vi "U3 Multiple EI-1050 Example.vi"() -> ()   [LabVIEW 2021]
panel:
  in  "stop":bool
  out "ms per iteration":u32
  out "RH B [%]":dbl format="%.6f"
  out "RH A [%]":dbl format="%.6f"
  out "Temp B [degC]":dbl format="%.6f"
  out "Temp A [degC]":dbl format="%.6f"
  out "Error Message":string
  out "error out":errorcluster
  # "Reads temperature and humidity from a pair of EI-1050 probes:\n\nBoth Probes:\nRed (Power)         FIO6\nBlack (Ground)     GND\nGreen (Data)        FIO4\nWhite (Clock)       FIO5\n\nProbe A:\nBrown (Enable)    FIO7\n\nProbe B:\nBrown (Enable)    DAC0"
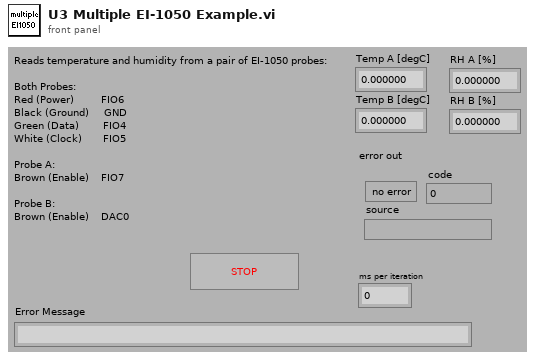
[diagram p1: front panel]
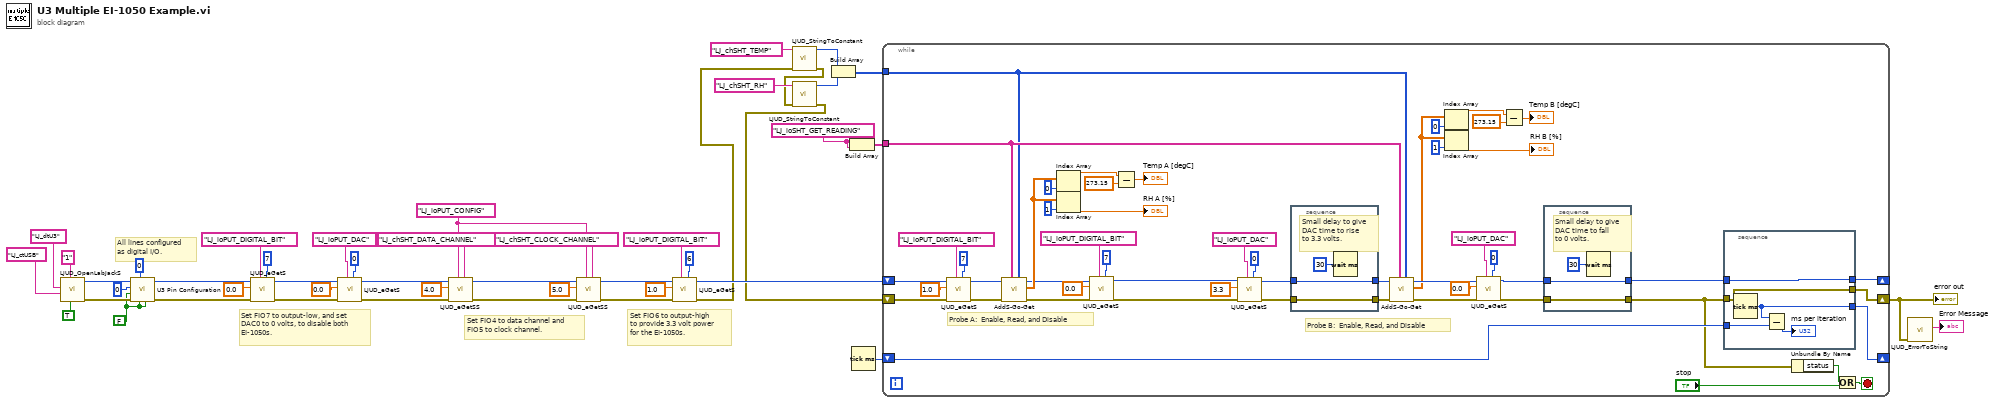
[diagram p0: block diagram]
diagram:
  w3 = "LJ_ioPUT_CONFIG"
  w39 = FALSE ("Enable DAC1")
  w34 = "LJ_ioSHT_GET_READING" ("IOType")
  # "Set FIO4 to data channel and\nFIO5 to clock channel."
  # "Set FIO7 to output-low, and set\nDAC0 to 0 volts, to disable both\nEI-1050s."
  # "Set FIO6 to output-high\nto provide 3.3 volt power\nfor the EI-1050s."
  # "All lines configured\nas digital I/O."
  n1 = call "LJUD_OpenLabJackS.vi"("FirstFound"=TRUE, "Address"="1", "ConnectionType"="LJ_ctUSB", "DeviceType"="LJ_dtU3") -> ("error out"=w41:errorcluster, "Handle"=w42:i32)  [unwired: 5 in, 1 out]
  n2 = call "U3 Pin Configuration.vi"("Enable Counter1"=w39, "Enable Counter0"=w39, "FIO/EIO Analog Enable"=0, "error in"=w41, "Enable DAC1"=w39, "Number of Timers Enabled"=u8 0, "Handle In"=w42) -> ("error out"=w20:errorcluster, "Handle Out"=w21:i32)  [unwired: 3 in]
  n3 = call "LJUD_eGetS.vi"("Channel"=7, "IOType"="LJ_ioPUT_DIGITAL_BIT", "error in"=w20, "Value Write"=0.0, "Handle In"=w21) -> ("error out"=w22:errorcluster, "Handle Out"=w23:i32)  [unwired: 4 in, 1 out]
  n4 = call "LJUD_eGetS.vi"("Channel"=0, "IOType"="LJ_ioPUT_DAC", "error in"=w22, "Value Write"=0.0, "Handle In"=w23) -> ("error out"=w5:errorcluster, "Handle Out"=w7:i32)  [unwired: 4 in, 1 out]
  n5 = call "LJUD_eGetSS.vi"("Channel"="LJ_chSHT_DATA_CHANNEL" ("IOType"), "IOType"=w3, "error in"=w5, "Value Write"=4.0, "Handle In"=w7) -> ("error out"=w11:errorcluster, "Handle Out"=w10:i32)  [unwired: 4 in, 1 out]
  n6 = call "LJUD_eGetSS.vi"("Channel"="LJ_chSHT_CLOCK_CHANNEL" ("IOType"), "IOType"=w3, "error in"=w11, "Value Write"=5.0, "Handle In"=w10) -> ("error out"=w4:errorcluster, "Handle Out"=w6:i32)  [unwired: 4 in, 1 out]
  n7 = call "LJUD_eGetS.vi"("Channel"=6, "IOType"="LJ_ioPUT_DIGITAL_BIT", "error in"=w4, "Value Write"=1.0, "Handle In"=w6) -> ("error out"=w14:errorcluster, "Handle Out"=w16:i32)  [unwired: 4 in, 1 out]
  n8 = call "LJUD_StringToConstant.vi"("error in"=w14, "String"="LJ_chSHT_TEMP") -> ("error out"=w13:errorcluster, "Constant Number"=w33:i32)  [unwired: 8 in]
  n9 = call "LJUD_StringToConstant.vi"("error in"=w13, "String"="LJ_chSHT_RH") -> ("error out"=w12:errorcluster, "Constant Number"=w32:i32)  [unwired: 8 in]
  n10 = Build Array(w33, w32) -> (w18:i32[])
  n11 = Build Array(w34, w34) -> (w19:string[])
  n12 = Tick Count (ms)() -> (millisecond timer value=w17:u32)
  n13 = while {
    shift-left: w17 -> [w59]
    shift-right: [w62] -> _
    shift-left: w16 -> [w63]
    shift-right: [w60] -> _
    shift-left: w12 -> [w64]
    shift-right: [w61] -> w15
    tunnel: w18 -> [w65]
    tunnel: w19 -> [w66]
    stop <- w58 stop-if-true
    # "Probe B:  Enable, Read, and Disable"
    # "Probe A:  Enable, Read, and Disable"
    n14 = call "LJUD_eGetS.vi"("Channel"=7, "IOType"="LJ_ioPUT_DIGITAL_BIT", "error in"=w64, "Value Write"=1.0, "Handle In"=w63) -> ("error out"=w89:errorcluster, "Handle Out"=w90:i32)  [unwired: 4 in, 1 out]
    n15 = call "AddS-Go-Get.vi"("Channels"=w65, "IOTypes"=w66, "error in"=w89, "Handle In"=w90) -> ("error out"=w84:errorcluster, "Values Read"=w98:dbl[], "Handle Out"=w85:i32)  [unwired: 5 in]
    n16 = Index Array(array=w98, index=0 ("Index")) -> (element=w95:dbl)
    n17 = Index Array(array=w98, index=1 ("Index")) -> (element=→"RH A [%]":dbl)
    n18 = call "LJUD_eGetS.vi"("Channel"=7, "IOType"="LJ_ioPUT_DIGITAL_BIT", "error in"=w84, "Value Write"=0.0, "Handle In"=w85) -> ("error out"=w69:errorcluster, "Handle Out"=w70:i32)  [unwired: 4 in, 1 out]
    n19 = Subtract(x=w95, y=273.15) -> (x-y=→"Temp A [degC]":dbl)
    n20 = call "LJUD_eGetS.vi"("Channel"=0, "IOType"="LJ_ioPUT_DAC", "error in"=w69, "Value Write"=3.3, "Handle In"=w70) -> ("error out"=w55:errorcluster, "Handle Out"=w53:i32)  [unwired: 4 in, 1 out]
    n21 = stacked-sequence {
      tunnel: w55 -> [w106]
      tunnel: [w106] -> w54
      tunnel: w53 -> [w105]
      tunnel: [w105] -> w52
      frame #0 {
        # "Small delay to give\nDAC time to rise\nto 3.3 volts."
        n22 = Wait (ms)(milliseconds to wait=u32 30) -> ()  [unwired: 1 out]
      }
    }
    n23 = call "AddS-Go-Get.vi"("Channels"=w65, "IOTypes"=w66, "error in"=w54, "Handle In"=w52) -> ("error out"=w83:errorcluster, "Values Read"=w73:dbl[], "Handle Out"=w82:i32)  [unwired: 5 in]
    n24 = Index Array(array=w73, index=0 ("Index")) -> (element=w75:dbl)
    n25 = Index Array(array=w73, index=1 ("Index")) -> (element=→"RH B [%]":dbl)
    n26 = call "LJUD_eGetS.vi"("Channel"=0, "IOType"="LJ_ioPUT_DAC", "error in"=w83, "Value Write"=0.0, "Handle In"=w82) -> ("error out"=w50:errorcluster, "Handle Out"=w51:i32)  [unwired: 4 in, 1 out]
    n27 = Subtract(x=w75, y=273.15) -> (x-y=→"Temp B [degC]":dbl)
    n28 = stacked-sequence {
      tunnel: w50 -> [w103]
      tunnel: [w103] -> w49
      tunnel: w51 -> [w102]
      tunnel: [w102] -> w48
      frame #0 {
        # "Small delay to give\nDAC time to fall\nto 0 volts."
        n29 = Wait (ms)(milliseconds to wait=u32 30) -> ()  [unwired: 1 out]
      }
    }
    n30 = stacked-sequence {
      tunnel: [w111] -> w62
      tunnel: w49 -> [w110]
      tunnel: [w110] -> w61
      tunnel: [w109] -> w60
      tunnel: w48 -> [w109]
      tunnel: w59 -> [w108]
      frame #0 {
        n31 = Tick Count (ms)() -> (millisecond timer value=w111:u32)
        n32 = Subtract(x=w111, y=w108) -> (x-y=→"ms per iteration":u32)
      }
    }
    n33 = Unbundle By Name(w49) -> ("status"=w57:bool)
    n34 = Or(x=w57, y="stop") -> (x .or. y?=w58:bool)
  }
  "error out" <- w15
  n35 = call "LJUD_ErrorToString.vi"("error in"=w15) -> ("String"=→"Error Message":string)  [unwired: 10 in]
